vi "G#RealTimeTemplate_CreateBase.vi"(0 "reference in":refnum<class "G#RealTimeTemplate.lvclass">, 5 "error in (no error)":errorcluster) -> (14 "reference out":refnum<class "G#RealTimeTemplate.lvclass">, 19 "error out":errorcluster)   [LabVIEW 2020, in "G#RealTimeTemplate.lvclass"]
doc: "Constructor."
uses:
  <vilib>/addons/_AddQ/G#Templates/G#RealTimeTemplate/G#RealTimeTemplate.lvclass
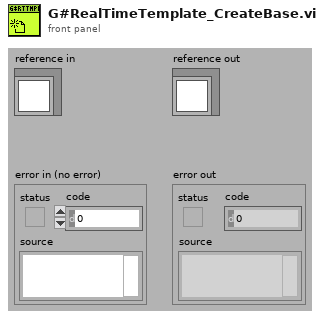
[diagram p1: front panel]
types:
  T1 = typedef "G#RealTimeTemplate.lvclass/ObjectAttributesRef.ctl" = refnum<data-value>
  T2 = typedef "G#RealTimeTemplate.lvclass/ObjectAttributes.ctl" = cluster{"MyAttribute":dbl}
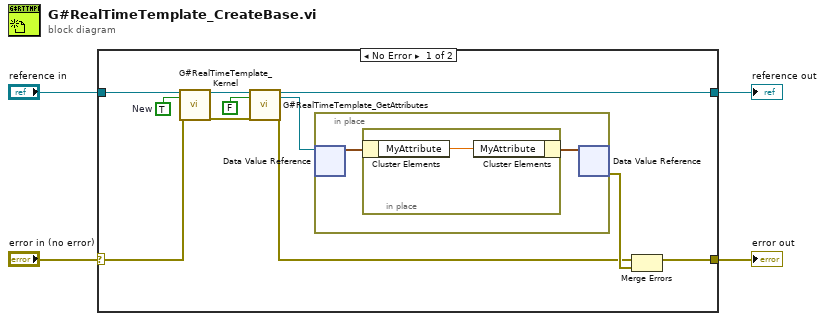
[diagram p0: block diagram]
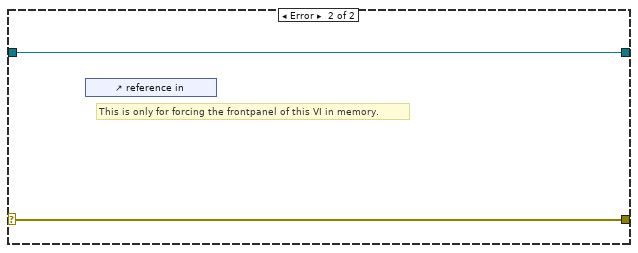
[diagram p2: hidden frame]
diagram:
  n1 = case shown="No Error" "error in (no error)" {
    selector: "error in (no error)" -> [w8 w20]
    tunnel: [w10 w20] -> w3
    tunnel: [w11 w19] -> w1
    tunnel: "reference in" -> [w9 w19]
    frame No Error {
      w5 = TRUE  # New
      n2 = call <vilib>:"G#RealTimeTemplate_Kernel.vi"("reference in"=w9, "New? (F=Dispose)"=w5, "error in (no error)"=w8) -> ("reference out"=w7:refnum<class "G#RealTimeTemplate.lvclass">, "error out"=w6:errorcluster)  [unwired: 15 in]
      n3 = call <vilib>:"G#RealTimeTemplate_GetAttributes.vi"("reference in"=w7, "return data? (T)"=FALSE ("return data"), "error in (no error)"=w6) -> ("reference out"=w11:refnum<class "G#RealTimeTemplate.lvclass">, "attributes ref"=w14:T1, "error out"=w12:errorcluster)  [unwired: 13 in, 1 out]
      n4 = in-place {
        n5 = in-place-dvr #1(w14) -> (w16:T2)  [unwired: 1 out]
        n6 = in-place {
          n7 = in-place-cluster #2(w16) -> ("MyAttribute"=w18:dbl)
          n8 = in-place-cluster #2("MyAttribute"=w18) -> (w17:T2)
        }
        n9 = in-place-dvr #1(w17) -> (w15:errorcluster)  [unwired: 1 out]
      }
      n10 = Merge Errors(w12, w15) -> (w10:errorcluster)
    }
    frame Error {
      # "This is only for forcing the frontpanel of this VI in memory."
      n11 = control-ref of="reference in"() -> ()  [unwired: 1 out]
    }
  }
  "error out" <- w3
  "reference out" <- w1
